vi "ReportStartBuild.vi"(0 "Table in":refnum<vi>, 1 "Operator":string, 2 "Numeric in":i32, 3 "ParametersVer":string, 4 "Consumer P/N":string, 5 "error in (no error)":errorcluster, 6 "SN":string, 7 "ApprovedBy":string, 8 "Tester Software Ver":string, 10 "P/N UUT":string) -> (14 "Numeric out":i32, 19 "error out":errorcluster)   [LabVIEW 2017]
uses:
  <vilib>/Utility/sysdir.llb/System Directory Type.ctl
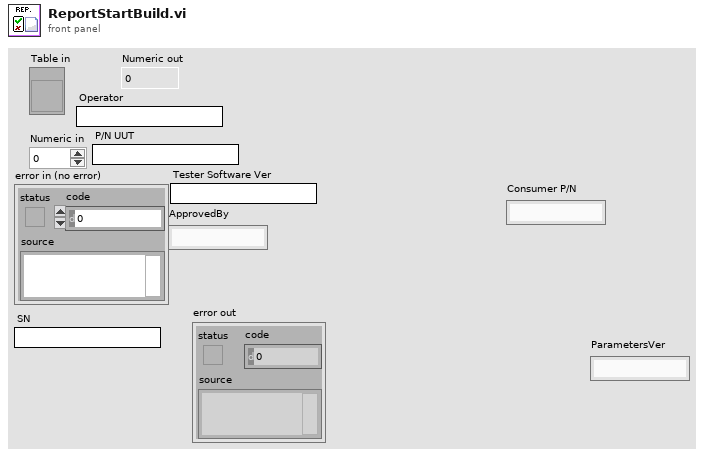
[diagram p1: front panel]
types:
  T1 = typedef "System Directory Type.ctl" = i32
  T2 = enum16{"open", "replace", "create", "open or create", "replace or create", "replace or create with confirmation"}
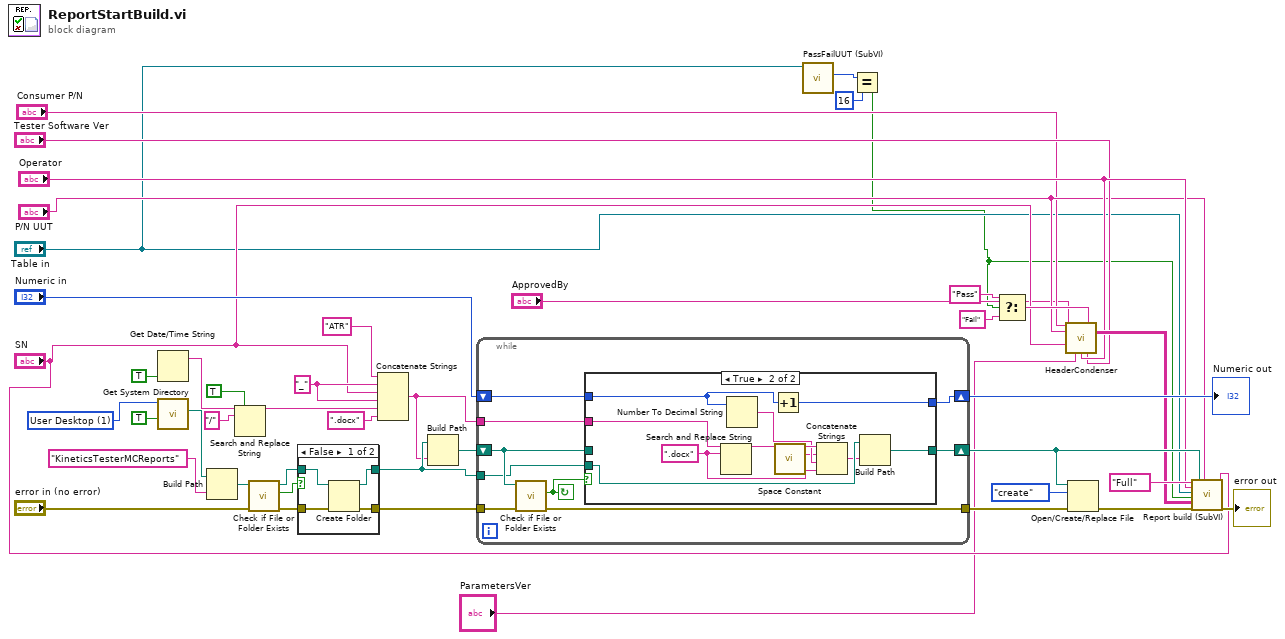
[diagram p0: block diagram]
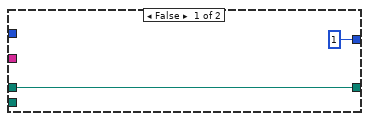
[diagram p2: hidden frame]
diagram:
  w40 = T1 1 items=["User Home"=0, "User Desktop"=1, "User Documents"=2, "User Application Data"=3, "User Preferences"=4, "User Temporary"=5, "Public Documents"=6, "Public Application Data"=7, "Public Preferences"=8, "Public Cache"=13, "System Core Libraries"=9, "System Installed Libraries"=10, "Application Files"=11, "Boot Volume Root"=12] ("system directory type")
  w43 = "_"
  n1 = Get Date/Time String(want seconds? (F)=TRUE) -> (date string=w22:string)  [unwired: 2 in, 1 out]
  n2 = call <vilib>:"Get System Directory.vi"("create directory if not found? (F)"=TRUE, "system directory type"=w40) -> ("system directory"=w41:path)  [unwired: 9 in]
  n3 = Build Path(base path=w41, name or relative path="KineticsTesterMCReports") -> (appended path=w24:path)
  n4 = Search and Replace String(replace all?=TRUE ("replace all? (F)"), input string=w22, search string="/") -> (result string=w33:string)  [unwired: 5 in, 3 out]
  n5 = call <vilib>:"Check if File or Folder Exists.vi"("error in (no error)"="error in (no error)", "path"=w24) -> ("error out"=w26:errorcluster, "file or folder exists?"=w23:bool, "dup path"=w25:path)  [unwired: 7 in]
  n6 = case shown="False" w23 {
    tunnel: w26 -> [w48 w49]
    tunnel: w25 -> [w47 w50]
    tunnel: [w46 w50] -> w38
    tunnel: [w45 w49] -> w44
    frame False {
      n7 = Create Folder(path (use dialog)=w47, error in=w48) -> (created path=w46:path, error out=w45:errorcluster)  [unwired: 1 in, 1 out]
    }
    frame True {
    }
  }
  n8 = Concatenate Strings("ATR" ("string"), w43, "SN", w43, w33, ".docx" ("string")) -> (w35:string)
  n9 = Build Path(base path=w38, name or relative path=w35) -> (appended path=w34:path)
  n10 = while {
    tunnel: w35 -> [w57]
    tunnel: w38 -> [w54]
    shift-right: [w56] -> w18
    shift-left: w34 -> [w55]
    shift-right: [w52] -> w37
    shift-left: "Numeric in" -> [w53]
    tunnel: w44 -> [w58]
    tunnel: [w59] -> w39
    stop <- w51 continue-if-true
    n11 = call <vilib>:"Check if File or Folder Exists.vi"("error in (no error)"=w58, "path"=w55) -> ("error out"=w59:errorcluster, "file or folder exists?"=w51:bool)  [unwired: 7 in, 1 out]
    n12 = case shown="True" w51 {
      tunnel: w57 -> [_ w71]
      tunnel: w53 -> [_ w63]
      tunnel: [w61 w68] -> w56
      tunnel: w55 -> [w61 _]
      tunnel: w54 -> [_ w69]
      tunnel: [1 w62] -> w52
      frame False {
      }
      frame True {
        w64 = ".docx" ("search string")
        n13 = Search and Replace String(input string=w71, search string=w64) -> (result string=w70:string)  [unwired: 6 in, 3 out]
        n14 = Number To Decimal String(number=w63) -> (decimal integer string=w66:string)  [unwired: 1 in]
        n15 = Increment(x=w63) -> (x+1=w62:i32)
        n16 = call <vilib>:"Space Constant.vi"() -> ("String"=w65:string)
        n17 = Concatenate Strings(w70, w65, w66, w64) -> (w67:string)
        n18 = Build Path(base path=w69, name or relative path=w67) -> (appended path=w68:path)
      }
    }
  }
  "Numeric out" <- w37
  n19 = call "PassFailUUT (SubVI).vi"("Table in"="Table in") -> ("Total Pass"=w3:i32)  [unwired: 8 in, 2 out]
  n20 = Equal?(x=w3, y=16) -> (x = y?=w1:bool)
  n21 = Select(t="Pass" ("y"), s=w1, f="Fail" ("y")) -> (s? t:f=w13:string)
  n22 = call "HeaderCondenser.vi"("Consumer P/N"="Consumer P/N", "GeneralResult"=w13, "P/N UUT"="P/N UUT", "ApprovedBy"="ApprovedBy", "Driver S/N"="SN", "Parameters Ver."="ParametersVer", "Oper."="Operator", "Tester Software Ver"="Tester Software Ver") -> ("Array"=w12:string[][])  [unwired: 6 in, 1 out]
  n23 = Open/Create/Replace File(file path (use dialog)=w18, error in=w39, operation (0:open)=T2."create") -> (error out=w17:errorcluster)  [unwired: 3 in, 2 out]
  n24 = call "Report build (SubVI).vi"("Full/Fails"="Full", "Operator"="Operator", "Original ATR Ref"="Table in", "GeneralResult-Pass(T)Fail(F)"=w1, "Header Array"=w12, "error in (no error)"=w17, "report file path"=w18, "PN"="P/N UUT", "SN"="SN") -> ("error out"=→"error out":errorcluster)  [unwired: 10 in]
